vi "PID.vi"(4 "Min Output":T1={"High"=100.0, "Low"=-100.0} {"Low" format="%#.8f"; "High" format="%#.8f"}, 5 "Max Output":T1={"High"=100.0, "Low"=-100.0} {"Low" format="%#.8f"; "High" format="%#.8f"}, 6 "Error I Zone":T1={"High"=10.0, "Low"=-10.0} {"Low" format="%#.8f"; "High" format="%#.8f"}, 7 "Acceptable Error":T1={"High"=0.1, "Low"=-0.1} {"Low" format="%#.8f"; "High" format="%#.8f"}, 8 "PID Gains":T2={"P"=1.0, "I"=0.01, "D"=0.0, "F"=0.0} {"F" format="%#.8f"; "D" format="%#.8f"; "I" format="%#.8f"; "P" format="%#.8f"}, 9 "Target Cycle Time(S)":dbl=0.05 format="%.3f", 10 "Setpoint":dbl format="%.2f", 11 "Process Variable":dbl format="%.2f") -> (0 "Time Mulitplyer Out":dbl, 1 "Error Out":dbl, 2 "PID Enabled Out":bool, 3 "Output Out":dbl format="%.2f")   [LabVIEW 2023]
uses:
  Shared Code/TypeDefs/Cluster_PID Gains.ctl
  Shared Code/TypeDefs/Cluster_High-Low.ctl
  <vilib>/addons/control/pid/NI_PID_pid.lvlib
  <vilib>/addons/control/pid/pid.llb/PID (DBL).vi
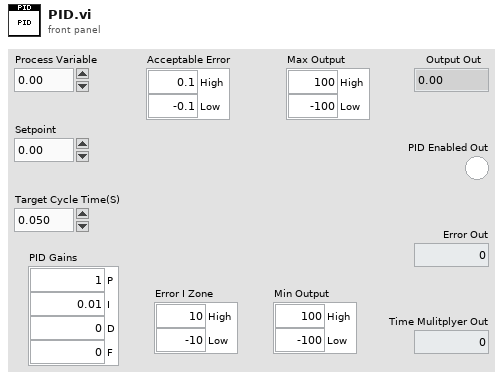
[diagram p1: front panel]
types:
  T1 = typedef "Cluster_High-Low.ctl" = cluster{"High":dbl, "Low":dbl}
  T2 = typedef "Cluster_PID Gains.ctl" = cluster{"P":dbl, "I":dbl, "D":dbl, "F":dbl}
  T3 = cluster{"PID gains":T2, "error":dbl, "process variable":dbl, "output ":dbl, "derivative action":dbl, "I Accumulator":dbl, "Previous Time":dbl, "Same Gains":bool, "time mulitplyer":dbl, "previous error":dbl, "Propotional Action":dbl, "Previous Process Value":dbl, "Acceptable Error":T1, "Error I Zone":T1, "Max output":T1, "Min Output":T1, "PID Enabled":bool}
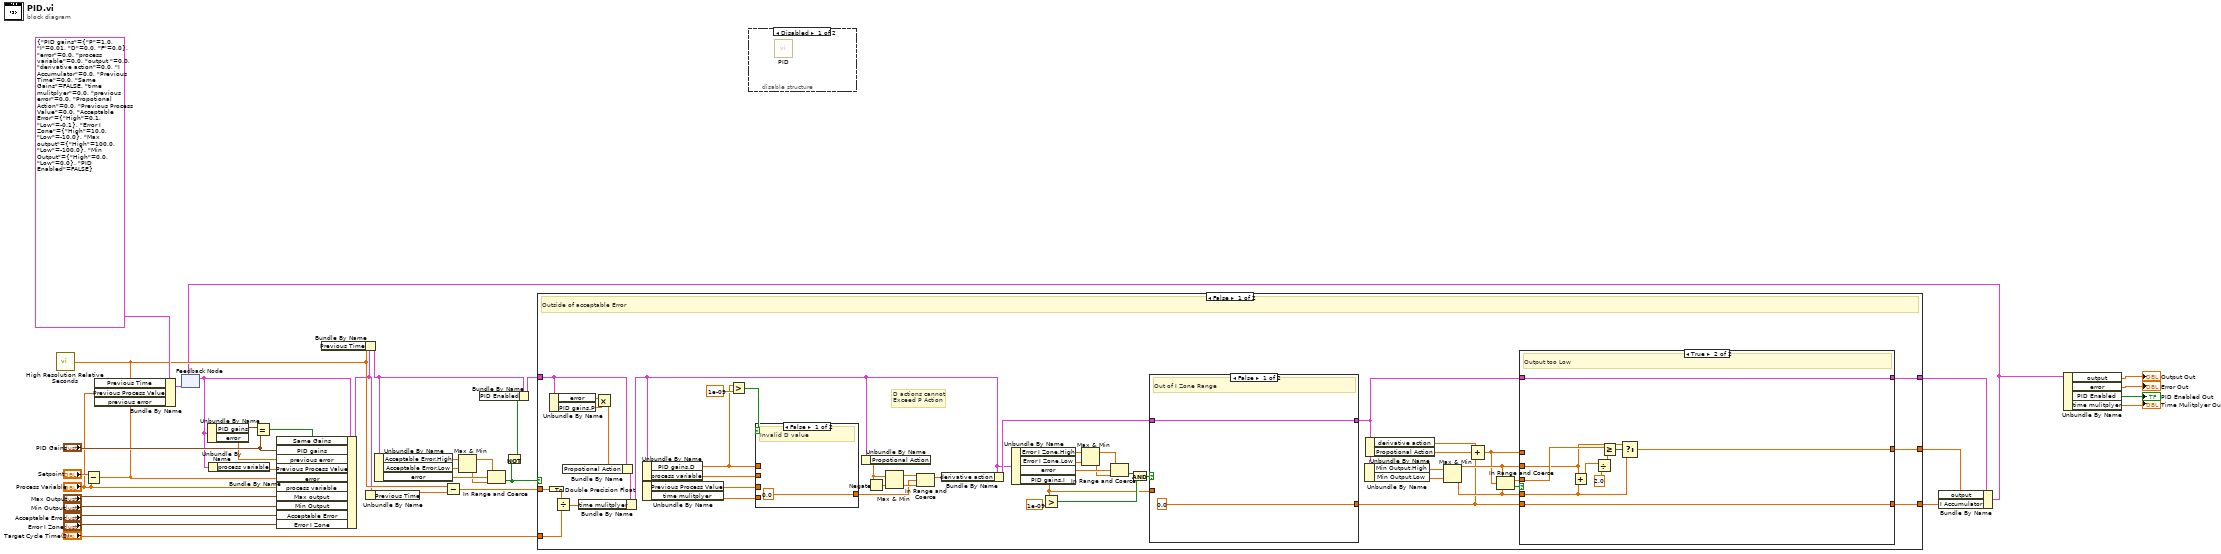
[diagram p0: block diagram]
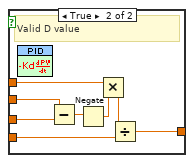
[diagram p2: hidden frame]
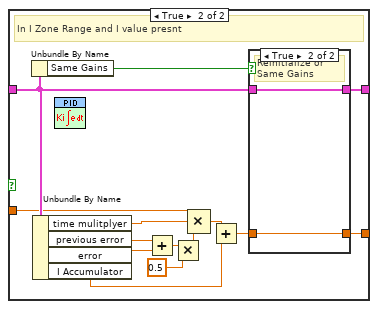
[diagram p3: hidden frame]
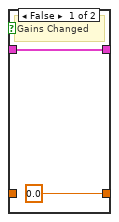
[diagram p4: hidden frame]
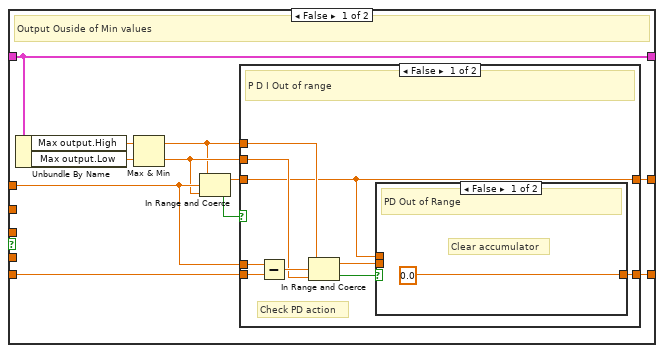
[diagram p5: hidden frame]
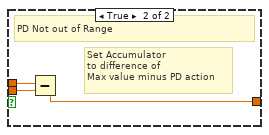
[diagram p6: hidden frame]
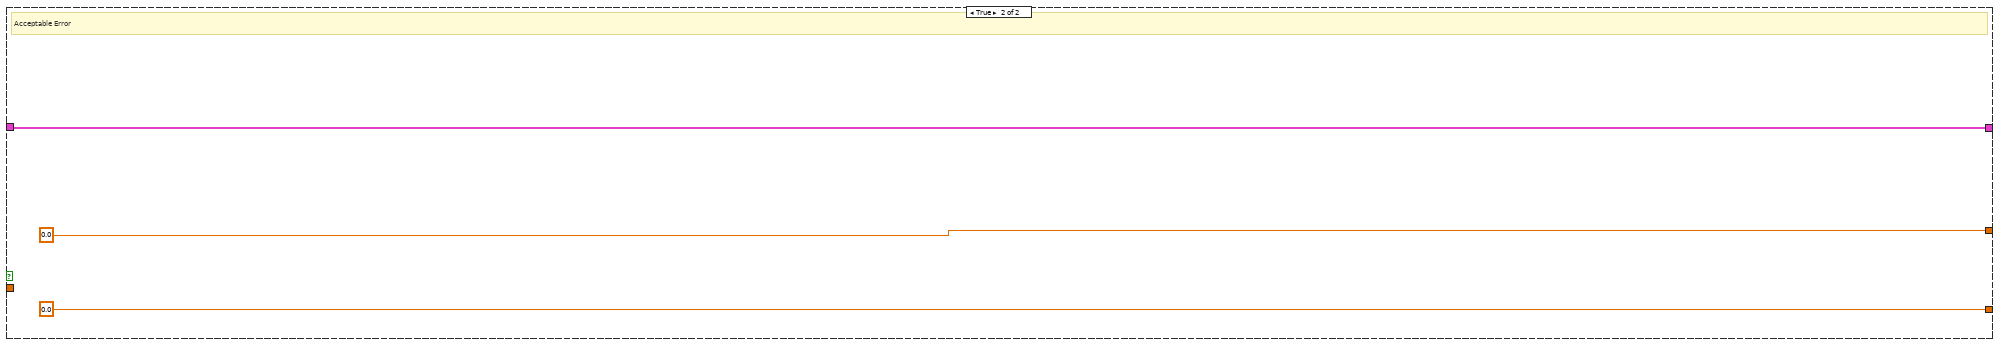
[diagram p8: hidden frame]
diagram:
  n1 = call <vilib>:"High Resolution Relative Seconds.vi"() -> ("relative seconds"=w32:dbl)
  n2 = Subtract(x="Setpoint", y="Process Variable") -> (x-y=w1:dbl)
  n3 = Bundle By Name(cluster=T3 {"PID gains"={"P"=1.0, "I"=0.01, "D"=0.0, "F"=0.0}, "error"=0.0, "process variable"=0.0, "output "=0.0, "derivative action"=0.0, "I Accumulator"=0.0, "Previous Time"=0.0, "Same Gains"=FALSE, "time mulitplyer"=0.0, "previous error"=0.0, "Propotional Action"=0.0, "Previous Process Value"=0.0, "Acceptable Error"={"High"=0.1, "Low"=-0.1}, "Error I Zone"={"High"=10.0, "Low"=-10.0}, "Max output"={"High"=100.0, "Low"=-100.0}, "Min Output"={"High"=0.0, "Low"=0.0}, "PID Enabled"=FALSE} ("Keep  Cluster"), "Previous Time"=w32, "Previous Process Value"="Process Variable", "previous error"=w1) -> (w5:T3)
  n4 = feedback #1(w5) -> (w4:T3)
  n5 = Unbundle By Name(w4) -> ("PID gains"=w23:T2, "error"=w21:dbl)
  n6 = Unbundle By Name(w4) -> ("process variable"=w18:dbl)
  n7 = Equal?(x=w23, y="PID Gains") -> (x = y?=w20:bool)
  n8 = Bundle By Name(cluster=w4, "Same Gains"=w20, "PID gains"="PID Gains", "previous error"=w21, "Previous Process Value"=w18, "error"=w1, "process variable"="Process Variable", "Max output"="Max Output", "Min Output"="Min Output", "Acceptable Error"="Acceptable Error", "Error I Zone"="Error I Zone") -> (w16:T3)
  n9 = Bundle By Name(cluster=w16, "Previous Time"=w32) -> (w9:T3)
  n10 = Unbundle By Name(w16) -> ("Previous Time"=w22:dbl)
  n11 = Unbundle By Name(w9) -> ("Acceptable Error.High"=w14:dbl, "Acceptable Error.Low"=w13:dbl, "error"=w15:dbl)
  n12 = Subtract(x=w32, y=w22) -> (x-y=w17:dbl)
  n13 = Max & Min(x=w14, y=w13) -> (max(x,y)=w11:dbl, min(x,y)=w12:dbl)
  n14 = In Range and Coerce(upper limit=w11, x=w15, lower limit=w12) -> (In Range?=w7:bool)  [unwired: 1 out]
  n15 = Not(x=w7) -> (.not. x?=w6:bool)
  n16 = Bundle By Name(cluster=w9, "PID Enabled"=w6) -> (w8:T3)
  n17 = case shown="False" w7 {
    tunnel: [w41 0.0] -> w24
    tunnel: [w57 w152] -> w19
    tunnel: "Target Cycle Time(S)" -> [w74 _]
    tunnel: w17 -> [w73 _]
    tunnel: w8 -> [w66 w152]
    tunnel: [w53 0.0 ("output")] -> w10
    frame False {
      # "D actions cannot\nExceed P Action"
      # "Outside of acceptable Error"
      n18 = To Double Precision Float(number=w73) -> (double precision float=w76:dbl)
      n19 = Unbundle By Name(w66) -> ("error"=w81:dbl, "PID gains.P"=w80:dbl)
      n20 = Divide(x=w76, y=w74) -> (x/y=w75:dbl)
      n21 = Multiply(x=w81, y=w80) -> (x*y=w77:dbl)
      n22 = Bundle By Name(cluster=w66, "Propotional Action"=w77) -> (w78:T3)
      n23 = Bundle By Name(cluster=w78, "time mulitplyer"=w75) -> (w48:T3)
      n24 = Unbundle By Name(w48) -> ("PID gains.D"=w49:dbl, "process variable"=w83:dbl)
      n25 = Unbundle By Name(w48) -> ("Previous Process Value"=w84:dbl, "time mulitplyer"=w82:dbl)
      n26 = Greater?(x=w49, y=1e-09) -> (0:w50:bool)
      n27 = case shown="False" w50 {
        tunnel: w84 -> [_ w91]
        tunnel: w82 -> [_ w90]
        tunnel: w83 -> [_ w88]
        tunnel: [0.0 w89] -> w43
        tunnel: w49 -> [_ w86]
        frame False {
          # "Invalid D value"
        }
        frame True {
          # "Valid D value"
          n28 = Subtract(x=w88, y=w91) -> (x-y=w93:dbl)
          n29 = Negate(x=w93) -> (-x=w87:dbl)
          n30 = Multiply(x=w86, y=w87) -> (x*y=w92:dbl)
          n31 = Divide(x=w92, y=w90) -> (x/y=w89:dbl)
        }
      }
      n32 = Unbundle By Name(w48) -> ("Propotional Action"=w47:dbl)
      n33 = Negate(x=w47) -> (-x=w46:dbl)
      n34 = Max & Min(x=w47, y=w46) -> (max(x,y)=w45:dbl, min(x,y)=w44:dbl)
      n35 = In Range and Coerce(upper limit=w45, x=w43, lower limit=w44) -> (coerced(x)=w42:dbl)  [unwired: 1 out]
      n36 = Bundle By Name(cluster=w48, "derivative action"=w42) -> (w79:T3)
      n37 = Unbundle By Name(w48) -> ("Error I Zone.High"=w65:dbl, "Error I Zone.Low"=w64:dbl, "error"=w72:dbl, "PID gains.I"=w67:dbl)
      n38 = Greater?(x=w67, y=1e-09) -> (0:w68:bool)
      n39 = Max & Min(x=w65, y=w64) -> (max(x,y)=w62:dbl, min(x,y)=w63:dbl)
      n40 = In Range and Coerce(upper limit=w62, x=w72, lower limit=w63) -> (In Range?=w71:bool)  [unwired: 1 out]
      n41 = And(x=w71, y=w68) -> (x .and. y?=w69:bool)
      n42 = case shown="False" w69 {
        tunnel: [0.0 w109] -> w39
        tunnel: [w95 w108] -> w40
        tunnel: w79 -> [w95 w107]
        tunnel: w67 -> [_ w98]
        frame False {
          # "Out of I Zone Range"
        }
        frame True {
          # "In I Zone Range and I value presnt"
          n43 = Unbundle By Name(w107) -> ("Same Gains"=w97:bool)
          n44 = Unbundle By Name(w107) -> ("time mulitplyer"=w104:dbl, "previous error"=w103:dbl, "error"=w102:dbl, "I Accumulator"=w96:dbl)
          n45 = Add(x=w103, y=w102) -> (x+y=w101:dbl)
          n46 = Multiply(x=w101, y=0.5) -> (x*y=w99:dbl)
          n47 = Compound Arithmetic op=MULTIPLY(w98, w104, w99) -> (w106:dbl)
          n48 = Add(x=w106, y=w96) -> (x+y=w105:dbl)
          n49 = case shown="True" w97 {
            tunnel: w105 -> [_ w113]
            tunnel: [0.0 w113] -> w109
            tunnel: w107 -> [w111 w112]
            tunnel: [w111 w112] -> w108
            frame False {
              # "Gains Changed"
            }
            frame True {
              # "Reinitialize or Same Gains"
            }
          }
        }
      }
      n50 = Unbundle By Name(w40) -> ("Min Output.High"=w38:dbl, "Min Output.Low"=w61:dbl)
      n51 = Unbundle By Name(w40) -> ("derivative action"=w59:dbl, "Propotional Action"=w60:dbl)
      n52 = Max & Min(x=w38, y=w61) -> (max(x,y)=w56:dbl, min(x,y)=w55:dbl)
      n53 = Compound Arithmetic op=ADD(w59, w60, w39) -> (w52:dbl)
      n54 = In Range and Coerce(upper limit=w56, x=w52, lower limit=w55) -> (coerced(x)=w54:dbl, In Range?=w58:bool)
      n55 = case shown="True" w58 {
        tunnel: w40 -> [w122 w149]
        tunnel: [w122 w149] -> w57
        tunnel: w56 -> [_ w143]
        tunnel: w55 -> [_ w142]
        tunnel: w54 -> [_ w146]
        tunnel: [w118 w140] -> w53
        tunnel: w52 -> [w116 _]
        tunnel: w39 -> [w117 w141]
        tunnel: [w120 w141] -> w41
        frame False {
          # "Output Ouside of Min values"
          n56 = Unbundle By Name(w122) -> ("Max output.High"=w124:dbl, "Max output.Low"=w123:dbl)
          n57 = Max & Min(x=w124, y=w123) -> (max(x,y)=w114:dbl, min(x,y)=w115:dbl)
          n58 = In Range and Coerce(upper limit=w114, x=w116, lower limit=w115) -> (coerced(x)=w119:dbl, In Range?=w121:bool)
          n59 = case shown="False" w121 {
            tunnel: [w127 w138] -> w120
            tunnel: w117 -> [w131 w138]
            tunnel: w119 -> [w126 w139]
            tunnel: [w126 w139] -> w118
            tunnel: w116 -> [w132 _]
            tunnel: w115 -> [w129 _]
            tunnel: w114 -> [w128 _]
            frame False {
              # "Check PD action"
              # "P D I Out of range"
              n60 = Subtract(x=w132, y=w131) -> (x-y=w130:dbl)
              n61 = In Range and Coerce(upper limit=w128, x=w130, lower limit=w129) -> (coerced(x)=w125:dbl, In Range?=w133:bool)
              n62 = case shown="False" w133 {
                tunnel: [0.0 w135] -> w127
                tunnel: w126 -> [_ w137]
                tunnel: w125 -> [_ w136]
                frame False {
                  # "Clear accumulator"
                  # "PD Out of Range"
                }
                frame True {
                  # "Set Accumulator\nto difference of \nMax value minus PD action"
                  # "PD Not out of Range"
                  n63 = Subtract(x=w137, y=w136) -> (x-y=w135:dbl)
                }
              }
            }
            frame True {
              # "P,D I Within Range"
            }
          }
        }
        frame True {
          # "Output too Low"
          n64 = Add(x=w143, y=w142) -> (x+y=w148:dbl)
          n65 = Divide(x=w148, y=2.0) -> (x/y=w145:dbl)
          n66 = Greater Or Equal?(x=w146, y=w145) -> (x >= y?=w144:bool)
          n67 = Select(t=w143, s=w144, f=w142) -> (s? t:f=w140:dbl)
        }
      }
    }
    frame True {
      # "Acceptable Error"
    }
  }
  n68 = disable-structure shown="Disabled" {
    frame Disabled {
      n69 = call-poly <vilib>:"PID.vi"() -> ()  [unwired: 10 in, 2 out]
    }
    frame Enabled {
    }
  }
  n70 = Bundle By Name(cluster=w19, "output"=w10, "I Accumulator"=w24) -> (w3:T3)
  n71 = feedback-in #1(w3) -> ()
  n72 = Unbundle By Name(w3) -> ("output"=→"Output Out":dbl, "error"=→"Error Out":dbl, "PID Enabled"=→"PID Enabled Out":bool, "time mulitplyer"=→"Time Mulitplyer Out":dbl)
